vi "Xylo_Essai_2.vi"() -> ()   [LabVIEW 2018]
uses:
  058e16a7-a325-4137-b798-67b3c3899a1f.vi
panel:
  in  "RESET Button":bool
  out "Notes jouees":u8[](array[numeric])
  in  "stop":bool
  out "Numeric":i32
  in  "Array":bool[](array[boolean])=[FALSE, FALSE, FALSE, FALSE, FALSE, FALSE, FALSE, FALSE]
  out "Messure Musicale":dbl(graph)
  in  "File Path Control 2":path
  in  "Save Button":bool
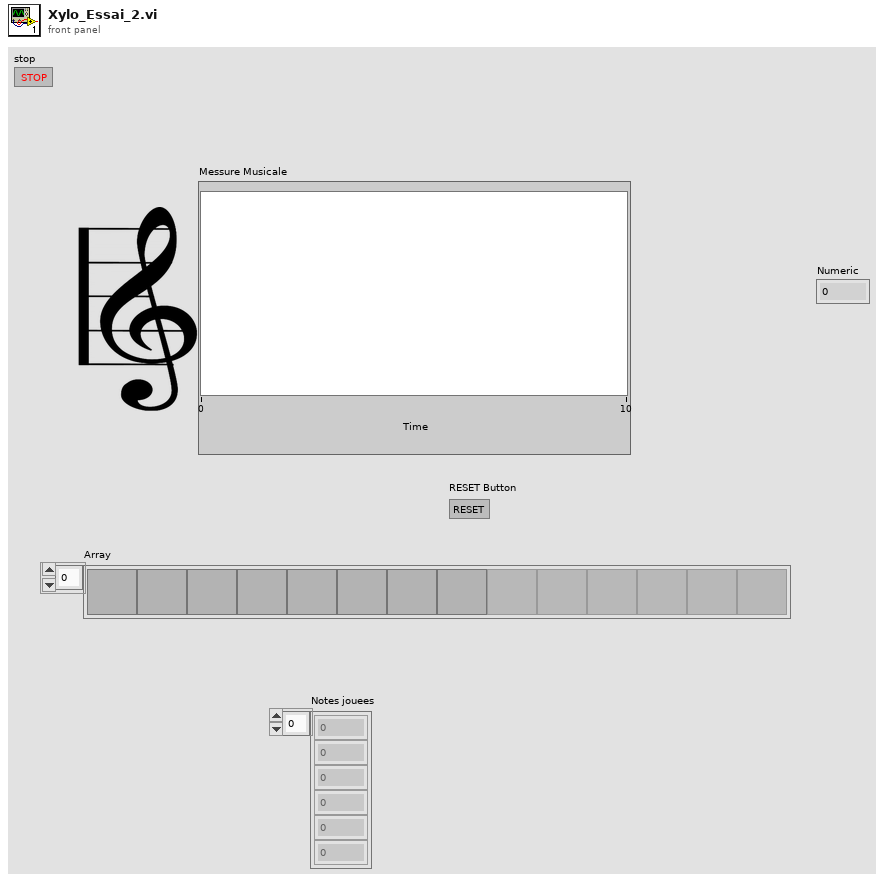
[diagram p1: front panel]
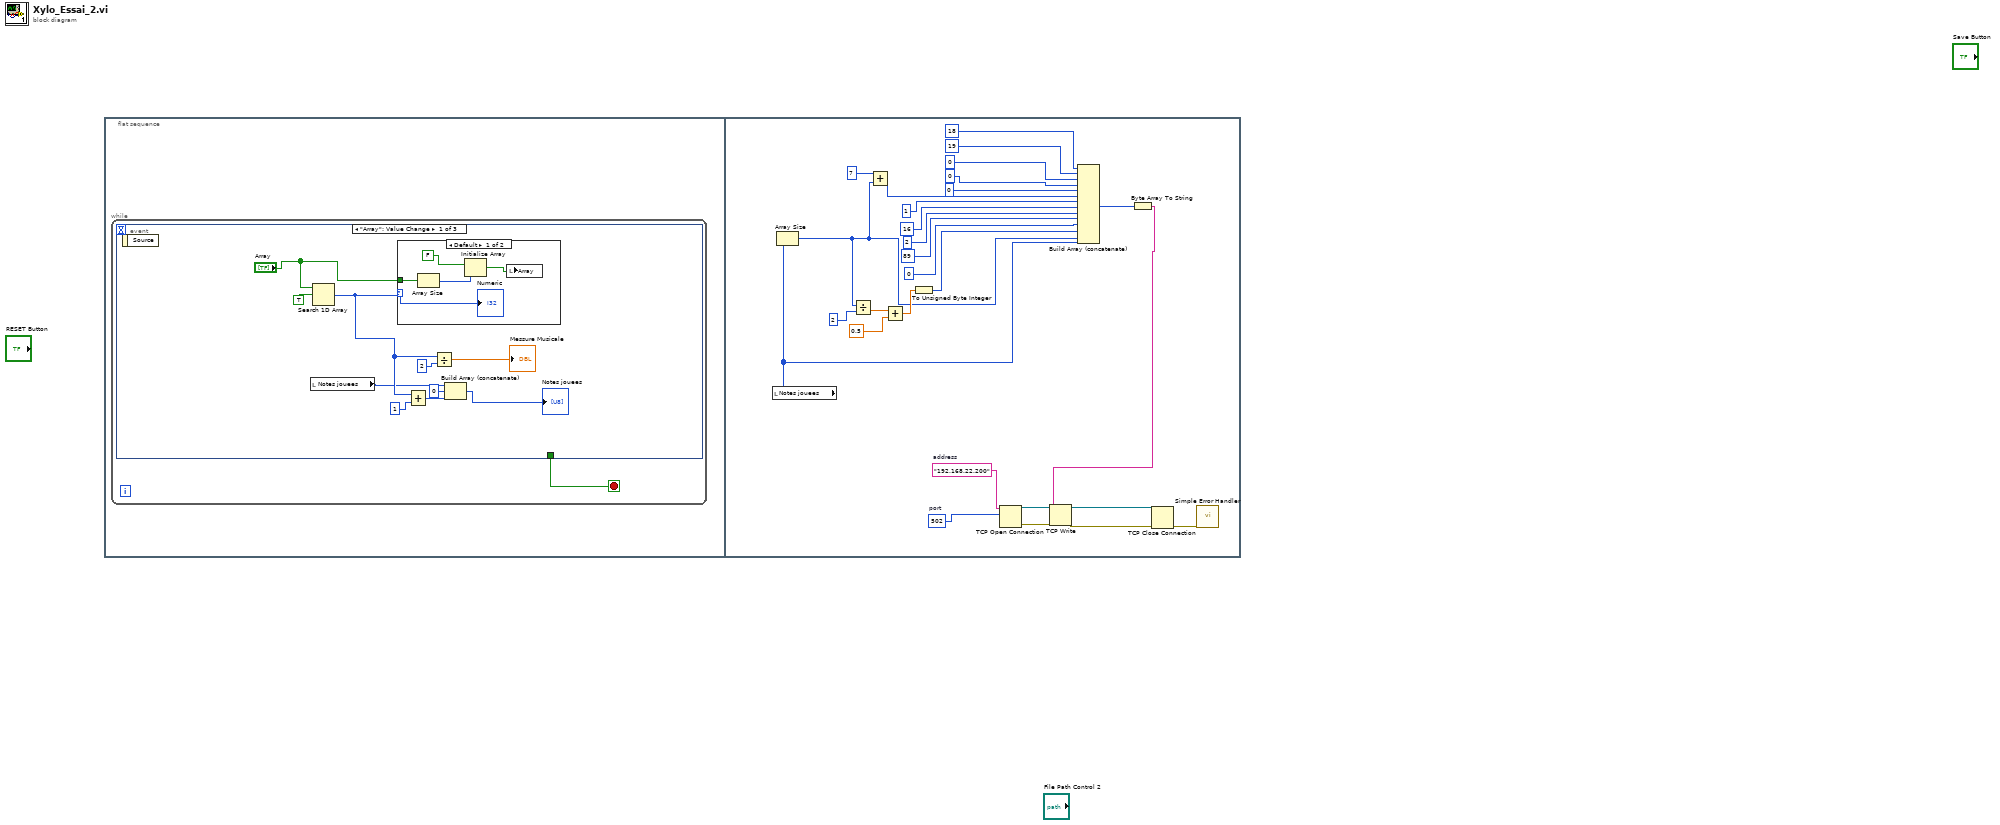
[diagram p0: block diagram]
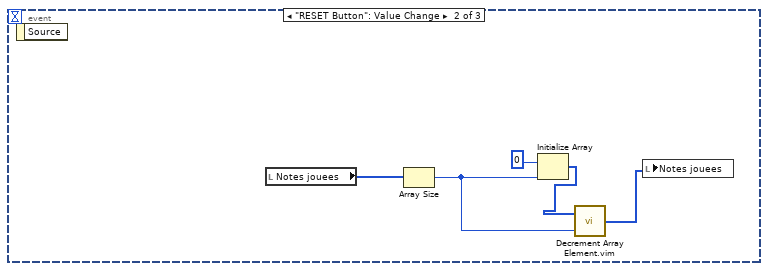
[diagram p3: hidden frame]
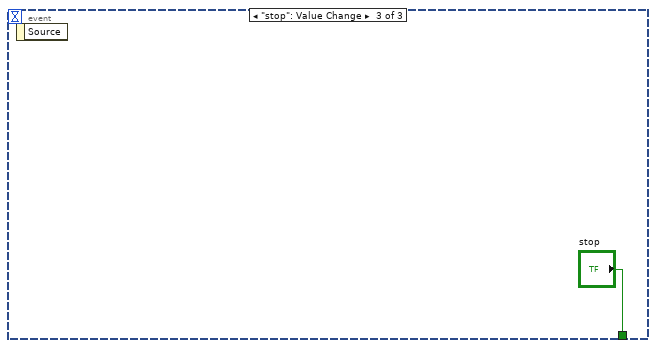
[diagram p4: hidden frame]
diagram:
  n1 = flat-sequence {
    frame #0 {
      n2 = while {
        stop <- w1 stop-if-true
        n3 = event shown="[0] \"Array\": Value Change" {
          selector: _ -> [_ _ _]
          dyn-events: _ -> [_ _ _]
          timeout: _ -> [_ _ _]
          tunnel: [_ _ "stop"] -> w1
          event "Array": Value Change {
            n4 = event-data() -> ()  [unwired: 1 in, 1 out]
            n5 = local read "Notes jouees"() -> (w5:u8[])
            n6 = Search 1D Array(1D array="Array", element=TRUE) -> (index of element=w7:i32)  [unwired: 1 in]
            n7 = case shown="Default" w7 {
              selector: w7 -> [w13 _]
              tunnel: "Array" -> [w14 _]
              frame Default {
                n8 = Array Size(array=w14) -> (size(s)=w16:i32)
                n9 = Initialize Array(FALSE ("element"), w16) -> (w12:bool[])
                n10 = local write "Array"(w12) -> ()
                "Numeric" <- w13
              }
              frame -1 {
              }
            }
            n11 = Add(x=w7, y=1) -> (x+y=w4:i32)
            n12 = Divide(x=w7, y=2 ("Numeric")) -> (x/y=→"Messure Musicale":dbl)
            n13 = Build Array (concatenate)(w5, 0 ("element"), w4) -> (→"Notes jouees":i32[])
          }
          event "RESET Button": Value Change {
            n14 = event-data() -> ()  [unwired: 1 in, 1 out]
            n15 = local read "Notes jouees"() -> (w20:u8[])
            n16 = Array Size(array=w20) -> (size(s)=w19:i32)
            n17 = Initialize Array(u8 0 ("element"), w19) -> (w18:u8[])
            n18 = call "Decrement Array Element.vim"("index"=w19, "array in"=w18) -> ("array out"=w17:u8[])
            n19 = local write "Notes jouees"(w17) -> ()
          }
          event "stop": Value Change {
            n20 = event-data() -> ()  [unwired: 1 in, 1 out]
          }
        }
      }
    }
    frame #1 {
      w35 = "192.168.22.200"  # address
      w36 = 502  # port
      n21 = local read "Notes jouees"() -> (w27:u8[])
      n22 = Array Size(array=w27) -> (size(s)=w24:i32)
      n23 = Divide(x=w24, y=2) -> (x/y=w25:dbl)
      n24 = Add(x=7, y=w24) -> (x+y=w50:i32)
      n25 = Add(x=w25, y=0.5) -> (x+y=w33:dbl)
      n26 = To Unsigned Byte Integer(number=w33) -> (unsigned 8bit integer=w28:u8)
      n27 = TCP Open Connection(address=w35, remote port or service name=w36) -> (connection ID=w49:refnum<k5>, error out=w48:errorcluster)  [unwired: 3 in]
      n28 = Build Array (concatenate)(18, 19, 0, 0, 0, w50, 1, 16, 2, 89, 0, w28, w24, w27) -> (w45:i32[])
      n29 = Byte Array To String(unsigned byte array=w45) -> (string=w44:string)
      n30 = TCP Write(connection ID=w49, data in=w44, error in (no error)=w48) -> (connection ID out=w46:refnum<k5>, error out=w47:errorcluster)  [unwired: 1 in, 1 out]
      n31 = TCP Close Connection(connection ID=w46, error in (no error)=w47) -> (error out=w43:errorcluster)  [unwired: 1 in, 1 out]
      n32 = call <vilib>:"Simple Error Handler.vi"("error in (no error)"=w43) -> ()  [unwired: 4 in, 5 out]
    }
  }
